vi "Index Array (String).vi"(8 "error in (no error)":errorcluster, 9 "index":i32, 10 "JSON Array in":refnum<class "JSON Array.lvclass">) -> (0 "error out":errorcluster, 1 "JSON String":refnum<class "JSON String.lvclass">)   [LabVIEW 2015, in "LVJSON.lvlib" / "JSON Array.lvclass"]
doc: "Returns the JSON String element of the JSON array at index."
uses:
  JSON Array.lvclass
  JSON String/JSON String.lvclass
  JSON Helper/To More Specific Type (String).vi
  JSON Helper/JSON Helper.lvclass
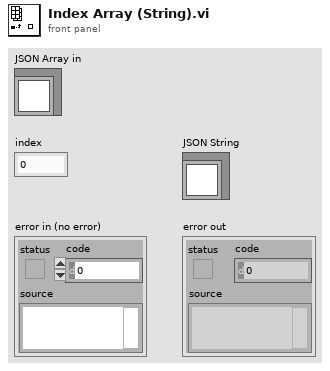
[diagram p1: front panel]
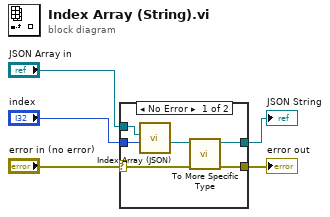
[diagram p0: block diagram]
diagram:
  n1 = case shown="No Error" "error in (no error)" {
    selector: "error in (no error)" -> [w8 w12]
    tunnel: [w7 w12] -> w4
    tunnel: "JSON Array in" -> [w10 _]
    tunnel: "index" -> [w11 _]
    tunnel: [w6 _] -> w1
    frame No Error {
      n2 = call "Index Array (JSON).vi"("index"=w11, "JSON Array in"=w10) -> ("JSON Data"=w9:refnum<class "JSON Null.lvclass">)  [unwired: 9 in]
      n3 = call-poly "To More Specific Type.vi"("error in (no error)"=w8, "JSON Datatype in"=w9) -> ("error out"=w7:errorcluster, "JSON Datatype out"=w6:refnum<class "JSON String.lvclass">)  [unwired: 8 in]
    }
    frame Error {
    }
  }
  "error out" <- w4
  "JSON String" <- w1
